vi "Scheduler hs.vi"(10 "Load Experimental Parameters":path, 11 "External Stop":refnum<vi>) -> ()   [LabVIEW 2019]
panel:
  out "EventData":string[][](array[string])
  out "doQueue1":refnum<queue>
  out "Event times":string[](array[string])
  out "current time":string
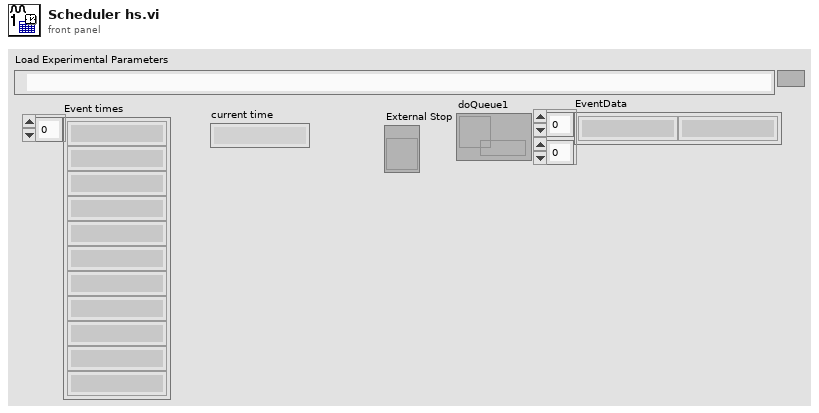
[diagram p1: front panel]
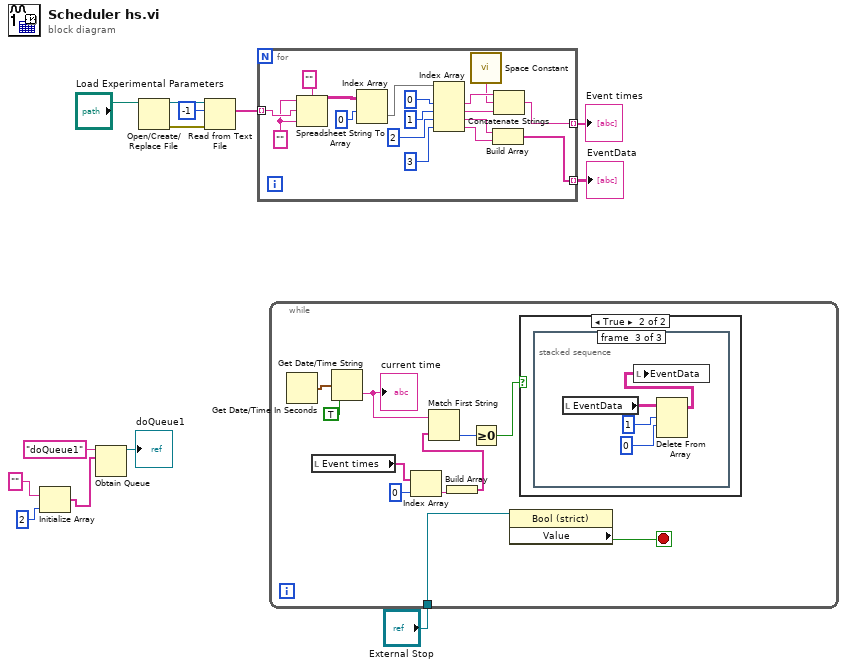
[diagram p0: block diagram]
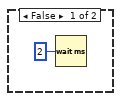
[diagram p2: hidden frame]
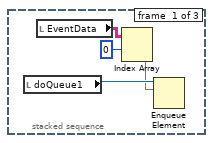
[diagram p3: hidden frame]
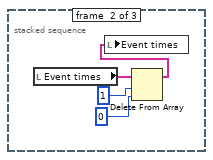
[diagram p4: hidden frame]
diagram:
  n1 = Initialize Array("", 2 ("dimension size")) -> (w5:string[])
  n2 = Obtain Queue(name (unnamed)="doQueue1", element data type=w5) -> (queue out=→"doQueue1":refnum<queue>)  [unwired: 3 in, 2 out]
  n3 = Open/Create/Replace File(file path (use dialog)="Load Experimental Parameters") -> (refnum out=w12:refnum<file>, error out=w11:errorcluster)  [unwired: 5 in, 1 out]
  n4 = Read from Text File(file (use dialog)=w12, count=-1, error in=w11) -> (text=w9:string[])  [unwired: 1 in, 3 out]
  n5 = for {
    tunnel: w9 -> [w29] mode=indexing
    tunnel: [w17] -> w8 mode=indexing
    tunnel: [w14] -> w1 mode=indexing
    w28 = "" ("format string")
    n6 = Spreadsheet String To Array(delimiter (Tab)="", format string=w28, spreadsheet string=w29, array type (2D Dbl)=w28) -> (array=w27:string[][])
    n7 = Index Array(array=w27, index (row)=0 ("disabled index (col)")) -> (element=w25:string[])  [unwired: 1 in]
    n8 = Index Array(array=w25, index #1=0 ("index"), index #2=1 ("index"), index #3=2 ("index"), index #4=3 ("index")) -> (element #1=w20:string, element #2=w19:string, element #3=w16:string, element #4=w15:string)
    n9 = call <vilib>:"Space Constant.vi"() -> ("String"=w18:string)
    n10 = Build Array(w16, w15) -> (w14:string[])
    n11 = Concatenate Strings(w20, w18, w19) -> (w17:string)
  }
  "Event times" <- w8
  "EventData" <- w1
  n12 = while {
    tunnel: "External Stop" -> [w35]
    stop <- w36 stop-if-true
    n13 = Get Date/Time In Seconds() -> (seconds since 1Jan1904=w41:timestamp)
    n14 = local read "Event times"() -> (w34:string[])
    n15 = Get Date/Time String(seconds (now)=w41, want seconds? (F)=TRUE) -> (time string=w39:string)  [unwired: 1 in, 1 out]
    "current time" <- w39
    n16 = Index Array(array=w34, index=0) -> (element=w32:string)
    n17 = Build Array(w32) -> (w31:string[])
    n18 = Match First String(2:w31, 3:w39) -> (0:w37:i32)  [unwired: 1 out]
    n19 = Greater Or Equal To 0?(x=w37) -> (x >= 0?=w38:bool)
    n20 = property class="Bool (strict)"(reference=w35) -> ("Value"=w36:bool)  [unwired: 1 in, 2 out]
    n21 = case shown="True" w38 {
      frame False {
        n22 = Wait (ms)(milliseconds to wait=u32 2) -> ()  [unwired: 1 out]
      }
      frame True {
        n23 = stacked-sequence {
          frame #0 {
            n24 = local read "doQueue1"() -> (w45:refnum<queue>)
            n25 = local read "EventData"() -> (w46:string[][])
            n26 = Index Array(array=w46, index (row)=0) -> (element=w44:string[])  [unwired: 1 in]
            n27 = Enqueue Element(queue=w45, element=w44) -> ()  [unwired: 2 in, 3 out]
          }
          frame #1 {
            n28 = local read "Event times"() -> (w48:string[])
            n29 = Delete From Array(array=w48, length=1, index=0) -> (array with subset deleted=w50:string[])  [unwired: 1 out]
            n30 = local write "Event times"(w50) -> ()
          }
          frame #2 {
            n31 = local read "EventData"() -> (w52:string[][])
            n32 = Delete From Array(array=w52, length=1, index (row)=0 ("index")) -> (array with subset deleted=w54:string[][])  [unwired: 1 in, 1 out]
            n33 = local write "EventData"(w54) -> ()
          }
        }
      }
    }
  }
